vi "Load Commands.vi"(8 "error in (no error)":errorcluster, 9 "Front (T) Back (F)":bool, 10 "Commands In":refnum<class "Command.lvclass">[](array[class]), 11 "Command Handler in":refnum<class "Command Handler.lvclass">) -> (0 "error out":errorcluster, 3 "Command Handler out":refnum<class "Command Handler.lvclass">)   [LabVIEW 2017, in "Command Handler.lvlib" / "Command Handler.lvclass"]
uses:
  Command Handler.lvclass
  Command Parents/Command.lvclass
  Command Handler.lvclass/Command Handler.ctl
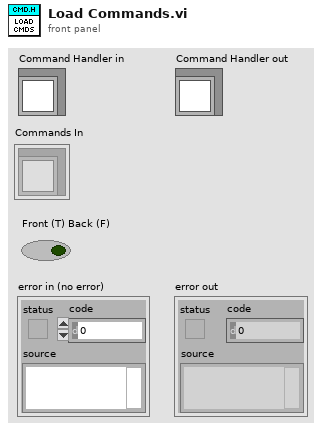
[diagram p1: front panel]
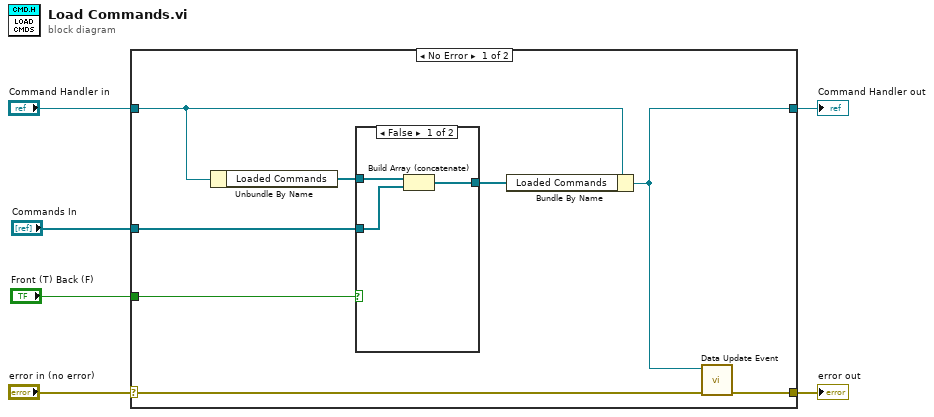
[diagram p0: block diagram]
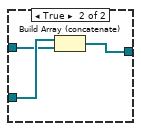
[diagram p2: hidden frame]
diagram:
  n1 = case shown="No Error" "error in (no error)" {
    selector: "error in (no error)" -> [w14 w22]
    tunnel: [w8 w22] -> w5
    tunnel: [w7 w21] -> w3
    tunnel: "Command Handler in" -> [w9 w21]
    tunnel: "Commands In" -> [w12 _]
    tunnel: "Front (T) Back (F)" -> [w11 _]
    frame No Error {
      n2 = Unbundle By Name(w9) -> ("Loaded Commands"=w13:refnum<class "Command.lvclass">[])
      n3 = case shown="False" w11 {
        tunnel: w13 -> [w17 w19]
        tunnel: w12 -> [w16 w20]
        tunnel: [w15 w18] -> w10
        frame False {
          n4 = Build Array (concatenate)(w17, w16) -> (w15:refnum<class "Command.lvclass">[])
        }
        frame True {
          n5 = Build Array (concatenate)(w20, w19) -> (w18:refnum<class "Command.lvclass">[])
        }
      }
      n6 = Bundle By Name(cluster=w9, "Loaded Commands"=w10) -> (w7:refnum<class "Command Handler.lvclass">)
      n7 = call "Data Update Event.vi"("error in (no error)"=w14, "Command Handler in"=w7) -> ("error out"=w8:errorcluster)  [unwired: 9 in]
    }
    frame Error {
    }
  }
  "error out" <- w5
  "Command Handler out" <- w3
